vi "MHM Write Params.vi"(8 "error in (no error)":errorcluster, 10 "ulVerify":u32, 11 "ulMHMHandle":u32) -> (0 "error out":errorcluster, 2 "pulValid":u32[](array[numeric]), 3 "function return":u32)   [LabVIEW 2019, in "MHM_1SL_interface.lvlib"]
uses:
  MHM_1SL_interface.lvlib
  lib/MHM_1SL_interface.dll
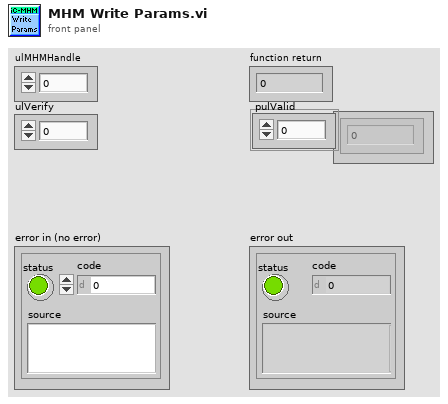
[diagram p1: front panel]
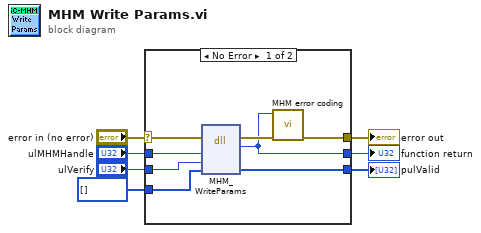
[diagram p0: block diagram]
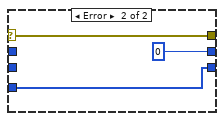
[diagram p2: hidden frame]
diagram:
  n1 = case shown="No Error" "error in (no error)" {
    selector: "error in (no error)" -> [w15 w18]
    tunnel: "ulMHMHandle" -> [w13 _]
    tunnel: "ulVerify" -> [w12 _]
    tunnel: [w11 w18] -> w4
    tunnel: [w10 u32 0 ("return type")] -> w3
    tunnel: [w9 w16] -> w1
    tunnel: u32[] [] ("pulValid") -> [w8 w16]
    frame No Error {
      n2 = dll-call lib="C:/workspace/project/scancon/MHM_1SL_interface_4.4.0/lv_interface/lib/MHM_1SL_interface.dll" fn="MHM_WriteParams"(error in=w15, "ulMHMHandle"=w13, "ulVerify"=w12, "pulValid"=w8) -> (error out=w14:errorcluster, "return type"=w10:u32, "pulValid"=w9:u32[])  [unwired: 4 in, 1 out]
      n3 = call "MHM error coding.vi"("error in (no error)"=w14, "function return in"=w10) -> ("error out"=w11:errorcluster)  [unwired: 9 in]
    }
    frame Error {
    }
  }
  "function return" <- w3
  "error out" <- w4
  "pulValid" <- w1
